vi "Destroy.vi"(8 "error in (no error)":errorcluster, 11 "ClientBase in":refnum<class "TCP.lvclass">) -> (0 "error out":errorcluster)   [LabVIEW 2020, in "TCP.lvlib" / "TCP.lvclass"]
uses:
  TCP.lvclass
  TCP.lvclass/TCP.ctl
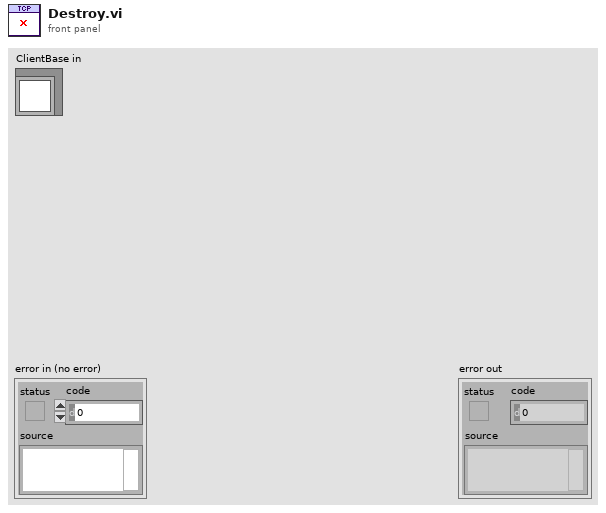
[diagram p1: front panel]
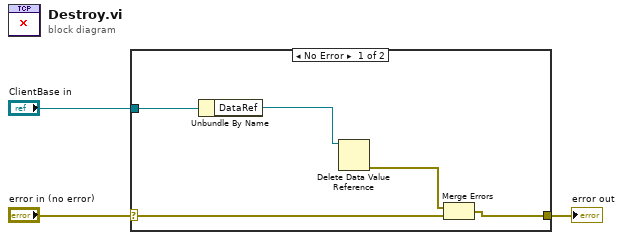
[diagram p0: block diagram]
diagram:
  n1 = case shown="No Error" "error in (no error)" {
    selector: "error in (no error)" -> [w8 w9]
    tunnel: [w5 w9] -> w2
    tunnel: "ClientBase in" -> [w7 _]
    frame No Error {
      n2 = Unbundle By Name(w7) -> ("DataRef"=w6:refnum<data-value>)
      n3 = Delete Data Value Reference(data value reference=w6) -> (error out=w4:errorcluster)  [unwired: 1 in, 1 out]
      n4 = Merge Errors(w4, w8) -> (w5:errorcluster)
    }
    frame Error {
    }
  }
  "error out" <- w2
